vi "Get object image.vi"() -> ()   [LabVIEW 2013]
panel:
  in  "Capturing window?":bool
  in  "Window/Control labels for Images ?":string[](array[string])
  in  "test VI Path":path=path "E:/Scrubbing/sceneWindowPick.vi"
  in  "Path to Auto test directory":path=path "C:/Perforce/user/inghoshr/Auto"
  in  "Create Folders?":bool
  out "error out":errorcluster
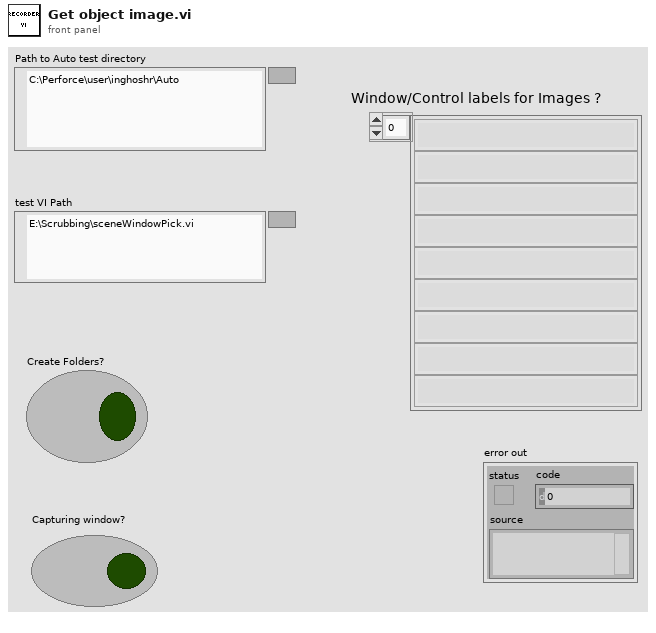
[diagram p1: front panel]
types:
  T1 = enum16{"open", "replace", "create", "open or create", "replace or create", "replace or create with confirmation"}
  T2 = cluster{"Window/Control labels for Images ?":string[], "Control Value:Get All":cluster{"Name":string, "Variant Data":variant}[]}
  T3 = typedef "imagedata.ctl" = cluster{"image type":i32, "image depth":i32, "image":u8[], "mask":u8[], "colors":u32[], "Rectangle":cluster{"left":i16, "top":i16, "right":i16, "bottom":i16}}
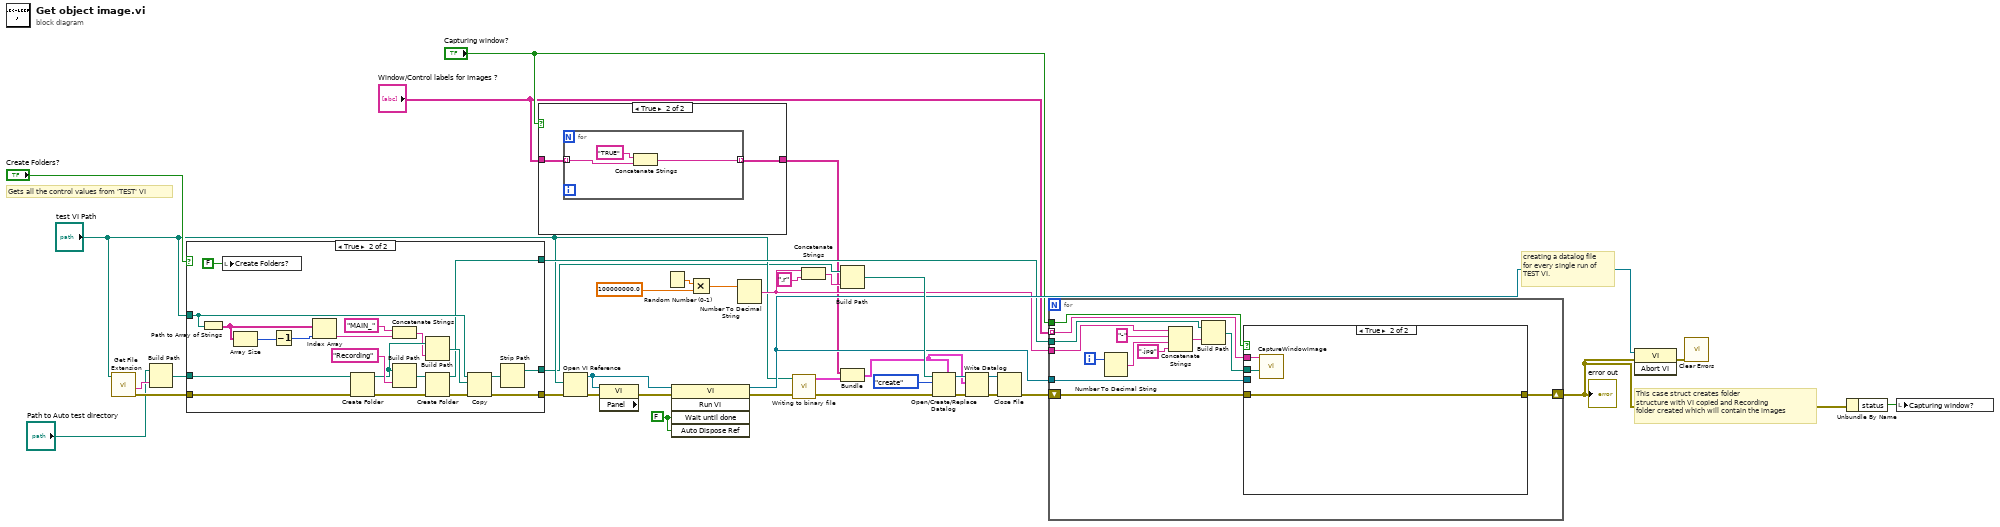
[diagram p0: block diagram]
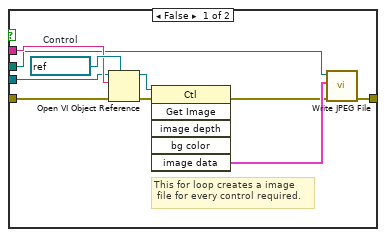
[diagram p3: hidden frame]
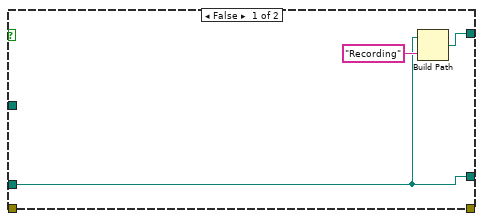
[diagram p4: hidden frame]
diagram:
  w5 = FALSE ("Wait Until Done")
  # "creating a datalog file \nfor every single run of\nTEST VI."
  # "Gets all the control values from 'TEST' VI"
  # "This case struct creates folder \nstructure with VI copied and Recording \nfolder created which will contain the images"
  n1 = call <vilib>:"Get File Extension.vi"("file"="test VI Path") -> ("error out"=w10:errorcluster, "filename without extension"=w12:string)  [unwired: 7 in, 2 out]
  n2 = Build Path(base path="Path to Auto test directory", name or relative path=w12) -> (appended path=w11:path)
  n3 = case shown="True" "Create Folders?" {
    tunnel: "test VI Path" -> [_ w55]
    tunnel: [w40 w50] -> w20
    tunnel: [_ w48] -> w36
    tunnel: w11 -> [w38 w47]
    tunnel: w10 -> [_ w46]
    tunnel: [w38 w44] -> w8
    frame False {
      n4 = Build Path(base path=w38, name or relative path="Recording") -> (appended path=w40:path)
    }
    frame True {
      n5 = Path to Array of Strings(0:w55) -> (2:w57:string[])  [unwired: 1 out]
      n6 = local write "Create Folders?"(FALSE ("Create Folders?")) -> ()
      n7 = Array Size(array=w57) -> (size(s)=w58:i32)
      n8 = Decrement(x=w58) -> (x-1=w56:i32)
      n9 = Index Array(array=w57, index=w56) -> (element=w43:string)
      n10 = Create Folder(path (use dialog)=w47, error in=w46) -> (created path=w53:path, error out=w52:errorcluster)  [unwired: 1 in, 1 out]
      n11 = Concatenate Strings("MAIN_" ("string"), w43) -> (w42:string)
      n12 = Build Path(base path=w53, name or relative path="Recording") -> (appended path=w60:path)
      n13 = Build Path(base path=w53, name or relative path=w42) -> (appended path=w54:path)
      n14 = Create Folder(path (use dialog)=w60, error in=w52) -> (created path=w50:path, error out=w51:errorcluster)  [unwired: 1 in, 1 out]
      n15 = Copy(8:w51, 10:w54, 11:w55) -> (0:w48:errorcluster, 3:w45:path)  [unwired: 2 in, 1 out]
      n16 = Strip Path(path=w45) -> (stripped path=w44:path)  [unwired: 1 out]
    }
  }
  n17 = case shown="True" "Capturing window?" {
    tunnel: "Window/Control labels for Images ?" -> [w61 w63]
    tunnel: [w61 w62] -> w3
    frame False {
    }
    frame True {
      n18 = for {
        tunnel: w63 -> [w66] mode=indexing
        tunnel: [w64] -> w62 mode=indexing
        n19 = Concatenate Strings("TRUE" ("string"), w66) -> (w64:string)
      }
    }
  }
  n20 = Open VI Reference(vi path="test VI Path", error in (no error)=w36) -> (vi reference=w37:refnum<vi>, error out=w34:errorcluster)  [unwired: 4 in]
  n21 = property class="VI" props=["Panel"](reference=w37, error in=w34) -> (error out=w19:errorcluster)  [unwired: 2 out]
  n22 = Random Number (0-1)() -> (number: 0 to 1=w33:dbl)
  n23 = invoke class="VI" method="Run VI"(reference=w37, error in=w19, "Wait until done"=w5, "Auto Dispose Ref"=w5) -> (reference out=w22:refnum<vi>, error out=w17:errorcluster)  [unwired: 1 in, 3 out]
  n24 = Multiply(x=w33, y=100000000.0) -> (x*y=w31:dbl)
  n25 = Number To Decimal String(number=w31) -> (decimal integer string=w21:string)  [unwired: 1 in]
  n26 = call "Writing to binary file.vi"("error in (no error)"=w17, "vi path"="test VI Path") -> ("error out"=w18:errorcluster, "Control Value:Get All"=w15:cluster{"Name":string, "Variant Data":variant}[])  [unwired: 2 in]
  n27 = Concatenate Strings(w21, ".r" ("string")) -> (w29:string)
  n28 = Build Path(base path=w8, name or relative path=w29) -> (appended path=w28:path)
  n29 = Bundle("Window/Control labels for Images ?"=w3, "Control Value:Get All"=w15) -> (w14:T2)  [unwired: 1 in]
  n30 = Open/Create/Replace Datalog(5:w14, 8:w18, 10:T1."create" ("operation (0:open)"), 11:w28) -> (0:w26:errorcluster, 3:w25:refnum<k1>)  [unwired: 2 in, 1 out]
  n31 = Write Datalog(4:w26, 6:w14, 7:w25) -> (0:w24:errorcluster, 3:w23:refnum<k1>)
  n32 = Close File(refnum=w23, error in=w24) -> (error out=w7:errorcluster)  [unwired: 1 out]
  n33 = for {
    tunnel: w20 -> [w70]
    shift-right: [w79] -> w2
    shift-left: w7 -> [w67]
    tunnel: "Window/Control labels for Images ?" -> [w68] mode=indexing
    tunnel: w22 -> [w78]
    tunnel: w21 -> [w71]
    tunnel: "Capturing window?" -> [w77]
    i -> [w72]
    n34 = Number To Decimal String(number=w72) -> (decimal integer string=w76:string)  [unwired: 1 in]
    n35 = Concatenate Strings(w71, "-" ("string"), w76, ".jpg" ("string")) -> (w74:string)
    n36 = Build Path(base path=w70, name or relative path=w74) -> (appended path=w69:path)
    n37 = case shown="True" w77 {
      tunnel: [w86 w92] -> w79
      tunnel: w68 -> [w85 w90]
      tunnel: w78 -> [w84 _]
      tunnel: w67 -> [w83 w92]
      tunnel: w69 -> [w80 w91]
      frame False {
        w89 = refnum<vi> refnum  # Control
        # "This for loop creates a image\n file for every control required."
        n38 = Open VI Object Reference(7:w89, 8:w83, 10:w85, 11:w84) -> (0:w82:errorcluster, 3:w88:refnum<vi>)
        n39 = invoke class="Ctl" method="Get Image"(reference=w88, error in=w82) -> (error out=w81:errorcluster, "image data"=w87:T3)  [unwired: 4 in, 4 out]
        n40 = call <vilib>:"Write JPEG File.vi"("error in (no error)"=w81, "image data"=w87, "path to JPEG file"=w80) -> ("error out"=w86:errorcluster)  [unwired: 7 in, 1 out]
      }
      frame True {
        n41 = call "CaptureWindowImage.vi"("File Path"=w91, "Window Name"=w90) -> ()  [unwired: 9 in, 1 out]
      }
    }
  }
  "error out" <- w2
  n42 = invoke class="VI" method="Abort VI"(reference=w22, error in=w2) -> (error out=w16:errorcluster)  [unwired: 1 in, 2 out]
  n43 = call <vilib>:"Clear Errors.vi"("error in (no error)"=w16) -> ()  [unwired: 6 in, 1 out]
  n44 = Unbundle By Name(w2) -> ("status"=w1:bool)
  n45 = local write "Capturing window?"(w1) -> ()
